vi "Mic_Init.vi"(6 "itteration":u32, 7 "# channels":u16, 8 "resolution":u16, 9 "Sample time":dbl, 10 "Sampling rate":u16, 11 "device":u16) -> (0 "error out":errorcluster, 3 "DAQ Prams":T2={"task ID"=0, "Num Pts"=0, "timeout"=0.0, "FIFO"=0, "Double Bounce"=1.0} {"Double Bounce" format="%#.2g"; "task ID" format="%.0x"})   [LabVIEW 2022 SP3]
uses:
  <vilib>/sound2/lvsound2.llb/Sound Input Task ID.ctl
  <vilib>/sound2/lvsound2.llb/Sampling Mode.ctl
  <vilib>/sound2/lvsound2.llb/Sound Data Format.ctl
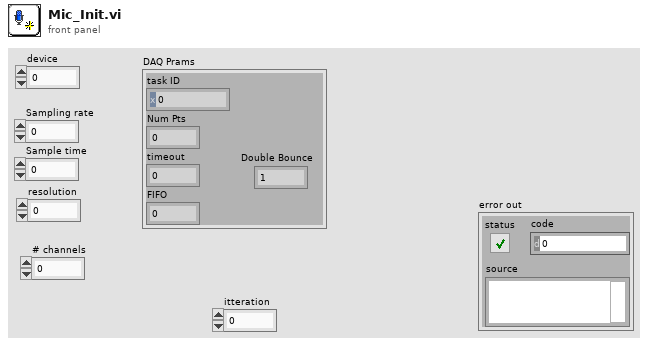
[diagram p1: front panel]
types:
  T1 = typedef "Sound Input Task ID.ctl" = u32
  T2 = cluster{"task ID":T1, "Num Pts":i32, "timeout":dbl, "FIFO":i32, "Double Bounce":dbl}
  T3 = cluster{"resolution":u16, "Sampling rate":u16, "Sample time":dbl, "device":u16, "# chan":u16}
  T4 = typedef "Sound Data Format.ctl" = cluster{"sample rate (S/s)":dbl, "number of channels":i32, "bits per sample":i32}
  T5 = typedef "Sampling Mode.ctl" = i32
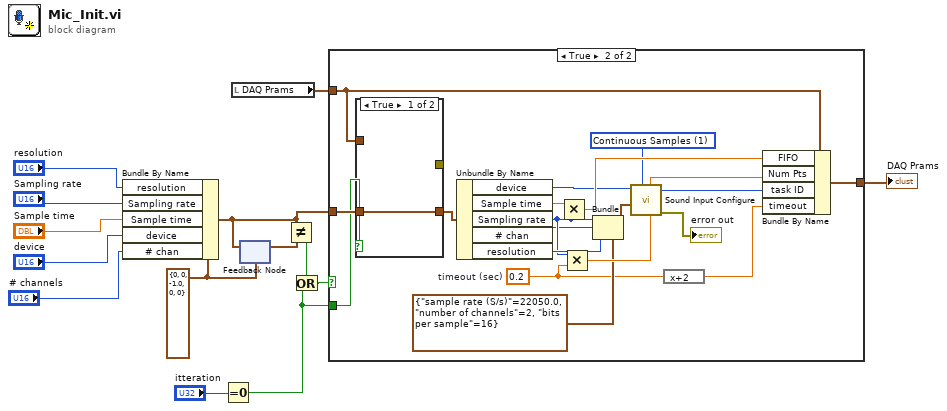
[diagram p0: block diagram]
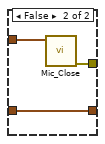
[diagram p3: hidden frame]
diagram:
  w11 = T3 {"resolution"=0, "Sampling rate"=0, "Sample time"=-1.0, "device"=0, "# chan"=0} ("settngs")
  n1 = Bundle By Name(cluster=w11, "resolution"="resolution", "Sampling rate"="Sampling rate", "Sample time"="Sample time", "device"="device", "# chan"="# channels") -> (w6:T3)
  n2 = Equal To 0?(x="itteration") -> (x = 0?=w2:bool)
  n3 = local read "DAQ Prams"() -> (w13:T2)
  n4 = feedback-in #1(w6) -> ()
  n5 = feedback #1(w11) -> (w12:T3)
  n6 = Not Equal?(x=w6, y=w12) -> (x != y?=w5:bool)
  n7 = Or(x=w5, y=w2) -> (x .or. y?=w3:bool)
  n8 = case shown="True" w3 {
    tunnel: [w15 w34] -> w14
    tunnel: w6 -> [_ w18]
    tunnel: w13 -> [w15 w20]
    tunnel: w2 -> [_ w17]
    frame False {
    }
    frame True {
      w24 = 0.2  # timeout (sec)
      w31 = T5 1 items=["Finite Samples", "Continuous Samples"] ("sample mode")
      n9 = case shown="True" w17 {
        tunnel: w20 -> [_ w38]
        tunnel: [w35 w37] -> w19
        tunnel: w18 -> [w35 w37]
        tunnel: [_ w36] -> _
        frame True {
        }
        frame False {
          n10 = call "Mic_Close.vi"("DAQ Prams"=w38) -> ("error out"=w36:errorcluster)  [unwired: 10 in]
        }
      }
      n11 = Unbundle By Name(w19) -> ("device"=w30:u16, "Sample time"=w27:dbl, "Sampling rate"=w25:u16, "# chan"=w16:u16, "resolution"=w26:u16)
      n12 = Multiply(x=w27, y=w25) -> (x*y=w32:dbl)
      n13 = Multiply(x=w25, y=w24) -> (x*y=w33:dbl)
      n14 = Bundle(cluster=T4 {"sample rate (S/s)"=22050.0, "number of channels"=2, "bits per sample"=16} ("sound format"), "sample rate (S/s)"=w25, "number of channels"=w16, "bits per sample"=w26) -> (w28:T4)
      n15 = call <vilib>:"Sound Input Configure.vi"("number of samples/ch"=w33, "sample mode"=w31, "sound format"=w28, "device ID"=w30) -> ("error out"=→"error out":errorcluster, "task ID"=w23:T1)  [unwired: 6 in]
      n16 = expression code="x+2"(w24) -> (w21:dbl)
      n17 = Bundle By Name(cluster=w20, "FIFO"=w32, "Num Pts"=w33, "task ID"=w23, "timeout"=w21) -> (w34:T2)
    }
  }
  "DAQ Prams" <- w14
